vi "Unit test-Optimal Motor Z start.vi"() -> ()   [LabVIEW 2017]
panel:
  out "FOVs in current cal":i32
  out "Points in current cal":i32
  in  "FOVs":i32[](array[numeric])=[175, 235, 350]
  in  "Previous cal":dbl[][](array[numeric])=[[148.1, 179.3, 262.9], [118.0, 140.7, 217.8], [90.0, 106.7, 183.1], [59.7, 68.6, 132.8], [27.9, 33.1, 74.0], [0.0, 0.0, 0.0], [-32.0, -50.0, -50.2], [-65.7, -90.6, -118.9], [-98.2, -135.6, -196.7], [-131.7, -182.8, -291.7], [-168.7, -223.8, -376.0]]
  out "Optimal motor Z start positions":dbl[](array[numeric])
  in  "New # cal points":i32=5
  in  "FOV info":cluster{"String":string, "Value":sgl}={"String"="175.5", "Value"=0.34}
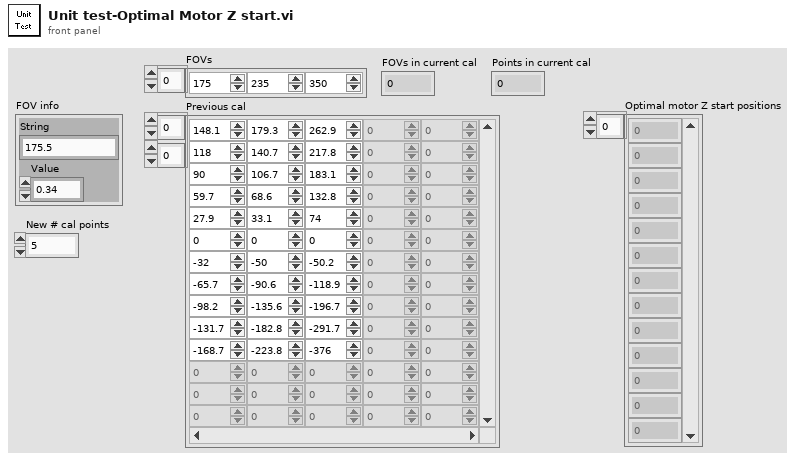
[diagram p1: front panel]
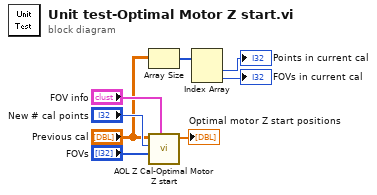
[diagram p0: block diagram]
diagram:
  n1 = Array Size(array="Previous cal") -> (size(s)=w2:i32[])
  n2 = call "AOL Z Cal-Optimal Motor Z start.vi"("FOV info"="FOV info", "FOVs"="FOVs", "Desired # cal points"="New # cal points", "Current Cal (no Norm Z column)"="Previous cal") -> ("Optimal motor Z start positions"=→"Optimal motor Z start positions":dbl[])  [unwired: 7 in]
  n3 = Index Array(array=w2) -> (element #1=→"Points in current cal":i32, element #2=→"FOVs in current cal":i32)  [unwired: 2 in]
